vi "Get Measurement Auto Range.vi"(0 "VISA resource name":refnum<visa-resource-name>, 11 "error in (no error)":errorcluster) -> (4 "VISA resource name out":refnum<visa-resource-name>, 6 "Voltage Auto Range Enabled?":bool, 8 "Current Auto Range Enabled?":bool, 10 "Resistance Auto Range Enabled?":bool, 15 "error out":errorcluster)   [LabVIEW 2020, in "Keithley 2450.lvlib"]
doc: "Gets whether the measurement auto range is enabled/disabled for V, I & R on the instrument."
uses:
  <instrlib>/Keithley 2450/Keithley 2450.lvlib
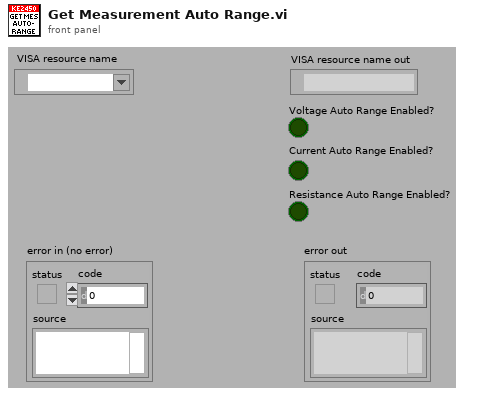
[diagram p1: front panel]
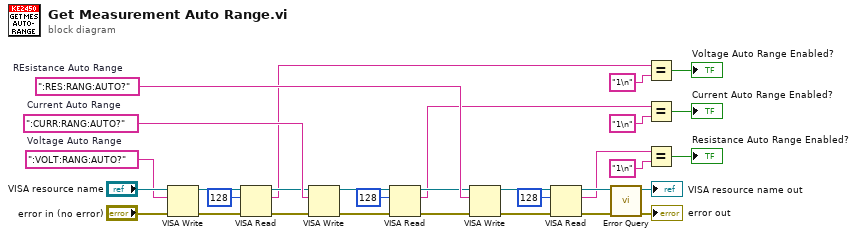
[diagram p0: block diagram]
diagram:
  w10 = ":RES:RANG:AUTO?"  # REsistance Auto Range
  w11 = ":CURR:RANG:AUTO?"  # Current Auto Range
  w12 = ":VOLT:RANG:AUTO?"  # Voltage Auto Range
  n1 = VISA Write(VISA resource name="VISA resource name", write buffer=w12, error in (no error)="error in (no error)") -> (VISA resource name out=w30:refnum<visa-resource-name>, error out=w31:errorcluster)  [unwired: 1 out]
  n2 = VISA Read(VISA resource name=w30, byte count=u32 128, error in (no error)=w31) -> (VISA resource name out=w8:refnum<visa-resource-name>, read buffer=w6:string, error out=w14:errorcluster)  [unwired: 1 out]
  n3 = VISA Write(VISA resource name=w8, write buffer=w11, error in (no error)=w14) -> (VISA resource name out=w22:refnum<visa-resource-name>, error out=w21:errorcluster)  [unwired: 1 out]
  n4 = VISA Read(VISA resource name=w22, byte count=u32 128, error in (no error)=w21) -> (VISA resource name out=w9:refnum<visa-resource-name>, read buffer=w5:string, error out=w15:errorcluster)  [unwired: 1 out]
  n5 = VISA Write(VISA resource name=w9, write buffer=w10, error in (no error)=w15) -> (VISA resource name out=w19:refnum<visa-resource-name>, error out=w20:errorcluster)  [unwired: 1 out]
  n6 = VISA Read(VISA resource name=w19, byte count=u32 128, error in (no error)=w20) -> (VISA resource name out=w7:refnum<visa-resource-name>, read buffer=w4:string, error out=w13:errorcluster)  [unwired: 1 out]
  n7 = call <instrlib>:"Error Query.vi"("error in (no error)"=w13, "VISA resource name"=w7) -> ("error out"=→"error out":errorcluster, "VISA resource name out"=→"VISA resource name out":refnum<visa-resource-name>)  [unwired: 8 out]
  n8 = Equal?(x=w6, y="1\n") -> (x = y?=→"Voltage Auto Range Enabled?":bool)
  n9 = Equal?(x=w5, y="1\n") -> (x = y?=→"Current Auto Range Enabled?":bool)
  n10 = Equal?(x=w4, y="1\n") -> (x = y?=→"Resistance Auto Range Enabled?":bool)
